vi "record_raw_data_FGV.vi"(7 "Mode":T1, 8 "error in":errorcluster, 11 "Parameter in":variant) -> (0 "error out":errorcluster, 3 "Parameter out":variant)   [LabVIEW 2016]
uses:
  Tools/three_modes.ctl
  MainFGV/cluster_main_FGV.ctl
  Config/Channel_config.ctl
  Config/test_config.ctl
  Config/feedType.ctl
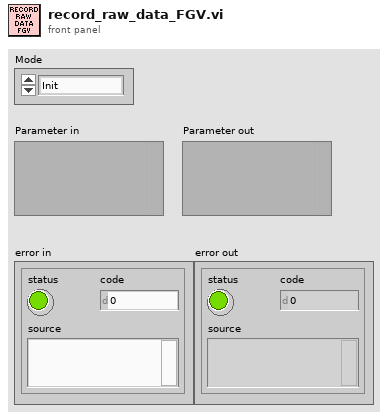
[diagram p1: front panel]
types:
  T1 = typedef "three_modes.ctl" = enum16{"Init", "Exec", "End"}
  T2 = typedef "cluster_main_FGV.ctl" = cluster{"Simulation?":bool, "ChanConfigs":T3[], "Test Config":T4, "Directory":path, "TestName":string, "RawFile":refnum<file>, "InfoFile":refnum<file>, "DataFile":refnum<file>, "task":refnum<k21>, "qRecord":refnum<queue>, "qProcess":refnum<queue>, "feed":T5}
  T3 = typedef "Channel_config.ctl" = cluster{"Canal":i32, "GF":dbl, "SC":bool}
  T4 = typedef "test_config.ctl" = cluster{"HoleDiam":dbl, "MeanLineDiam":dbl, "IncF":dbl, "ElastMod":dbl, "PoissonMod":dbl, "RosType":enum16{"Tipo A", "Tipo B", "Tipo C"}, "Método de análise":enum16{"Não uniforme 2013", "Simplificado 2013", "Simplificado 2008"}, "Pfinal":dbl, "AStop":bool}
  T5 = typedef "feedType.ctl" = enum16{"Manual", "Automático"}
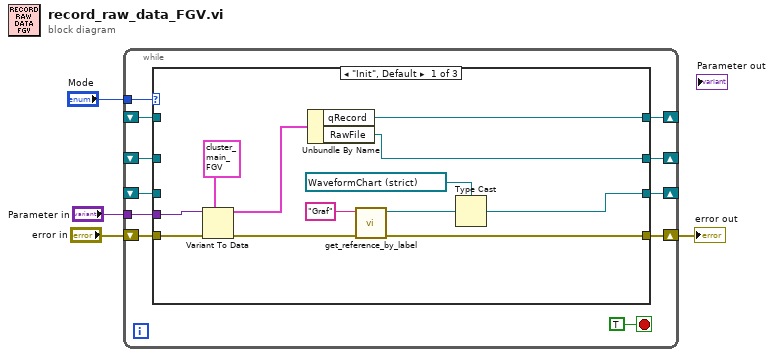
[diagram p0: block diagram]
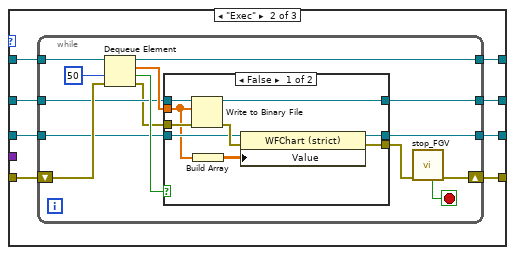
[diagram p2: hidden frame]
diagram:
  n1 = while {
    tunnel: "Mode" -> [w14]
    tunnel: "Parameter in" -> [w12]
    shift-right: [w10] -> w1
    shift-left: "error in" -> [w13]
    shift-right: [w11] -> _
    shift-left: _ -> [w9]
    shift-right: [w8] -> _
    shift-left: _ -> [w7]
    shift-right: [w6] -> _
    shift-left: _ -> [w5]
    stop <- TRUE stop-if-true
    n2 = case shown="\"Init\", Default" w14 {
      tunnel: w13 -> [w25 w35 w62]
      tunnel: w12 -> [w27 _ _]
      tunnel: [w22 w32 _] -> w11
      tunnel: [w19 w34 w62] -> w10
      tunnel: w9 -> [_ w33 _]
      tunnel: [w23 w30 _] -> w8
      tunnel: w7 -> [_ w31 _]
      tunnel: [w16 w28 _] -> w6
      tunnel: w5 -> [_ w29 _]
      frame "Init", Default {
        n3 = Variant To Data(error in=w25, type=T2 {"Simulation?"=FALSE, "ChanConfigs"=[], "Test Config"={"HoleDiam"=1.4, "MeanLineDiam"=5.0, "IncF"=0.2, "ElastMod"=207.0, "PoissonMod"=0.3, "RosType"=enum."Tipo A", "Método de análise"=enum."Simplificado 2008", "Pfinal"=0.3, "AStop"=TRUE}, "Directory"=path "", "TestName"="", "RawFile"=refnum, "InfoFile"=refnum, "DataFile"=refnum, "task"="", "qRecord"=refnum, "qProcess"=refnum, "feed"=enum."Manual"} ("cluster_main_FGV"), Variant=w27) -> (data=w24:T2, error out=w20:errorcluster)
        n4 = Unbundle By Name(w24) -> ("qRecord"=w23:refnum<queue>, "RawFile"=w22:refnum<file>)
        n5 = call "get_reference_by_label.vi"("error in"=w20, "Label"="Graf") -> ("error out"=w19:errorcluster, "Ctl Refnum"=w18:refnum<vi>)  [unwired: 7 in, 1 out]
        n6 = Type Cast(type=refnum<vi> refnum ("Graf"), x=w18) -> (*(type *) &x=w16:refnum<vi>)
      }
      frame "Exec" {
        n7 = while {
          shift-right: [w48] -> w34
          shift-left: w35 -> [w46]
          tunnel: w33 -> [w41]
          tunnel: [w38] -> w32
          tunnel: w31 -> [w47]
          tunnel: [w43] -> w30
          tunnel: w29 -> [w37]
          tunnel: [w36] -> w28
          stop <- w49 stop-if-true
          n8 = Dequeue Element(queue=w47, timeout in ms (-1)=50, error in (no error)=w46) -> (queue out=w43:refnum<queue>, element=w42:dbl[], timed out?=w44:bool, error out=w40:errorcluster)
          n9 = case shown="False" w44 {
            tunnel: w42 -> [w51 _]
            tunnel: w41 -> [w58 w61]
            tunnel: w40 -> [w57 w60]
            tunnel: [w54 w60] -> w39
            tunnel: [w56 w61] -> w38
            tunnel: w37 -> [w53 w59]
            tunnel: [w52 w59] -> w36
            frame False {
              n10 = Write to Binary File(file (use dialog)=w58, data=w51, error in=w57) -> (refnum out=w56:refnum<file>, error out=w55:errorcluster)  [unwired: 3 in, 1 out]
              n11 = Build Array(w51) -> (w50:dbl[][])
              n12 = property class="WFChart (strict)"(reference=w53, error in=w55, "Value"=w50) -> (reference out=w52:refnum<vi>, error out=w54:errorcluster)
            }
            frame True {
            }
          }
          n13 = call "stop_FGV.vi"("error in (no error)"=w39) -> ("error out"=w48:errorcluster, "parar?"=w49:bool)  [unwired: 9 in]
        }
      }
      frame "End" {
      }
    }
  }
  "error out" <- w1
